vi "Scale Values.vi"(0 "input variable":dbl, 5 "input min":dbl, 7 "input max":dbl, 9 "output min":dbl, 11 "output max":dbl) -> (6 "output variable":dbl)   [LabVIEW 2014]
doc: "Takes one set of values and changes their range.\n\nEx: If a range is 0 - 100, it will change it to 0-180 if given correct values to terminals"
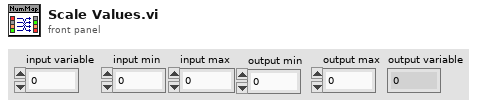
[diagram p1: front panel]
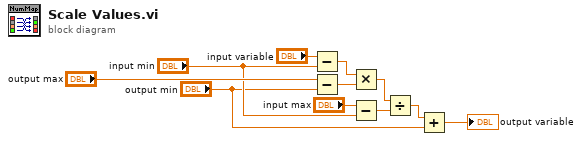
[diagram p0: block diagram]
diagram:
  n1 = Subtract(x="input variable", y="input min") -> (x-y=w8:dbl)
  n2 = Subtract(x="output max", y="output min") -> (x-y=w9:dbl)
  n3 = Multiply(x=w8, y=w9) -> (x*y=w5:dbl)
  n4 = Subtract(x="input max", y="input min") -> (x-y=w4:dbl)
  n5 = Divide(x=w5, y=w4) -> (x/y=w3:dbl)
  n6 = Add(x=w3, y="output min") -> (x+y=→"output variable":dbl)
